vi "CTRE_CANTalonSRX_GetPID.vi"(0 "CAN Talon SRX Ref":T1={"DeviceStatus"={"status"=FALSE, "code"=0, "source"=""}, "Type"=enum."PWM", "PWM"={"PWM Channel"=enum."PWM 1", "DeadBand"={"Name"="", "maxPositivePwm"=0, "minPositivePwm"=0, "centerPwm"=0, "maxNegativePwm"=0, "minNegativePwm"=0, "angularRange"=0}}, "CAN"={"Device Number"=0, "SetOutput VI Ref"=variant(enum8{"Percent VBus", "Current", "Speed", "Position", "Voltage"} enum."Percent VBus"), "GetOutput VI Ref"=variant(refnum<k1> refnum), "Enable VI Ref"=variant(dbl 12.0), "Disable VI Ref"=variant(enum8{"Percent VBus", "Speed", "Position", "Slave", "Unchanged / Invalid", "Voltage Compensation", "Current", "Motion Profile"} enum."Percent VBus"), "Data"=variant}, "Invert"=FALSE}, 1 "Parameter Slot":u8 max=1, 11 "error in (no error)":errorcluster) -> (4 "CAN Talon SRX Ref":T1={"DeviceStatus"={"status"=FALSE, "code"=0, "source"=""}, "Type"=enum."PWM", "PWM"={"PWM Channel"=enum."PWM 1", "DeadBand"={"Name"="", "maxPositivePwm"=0, "minPositivePwm"=0, "centerPwm"=0, "maxNegativePwm"=0, "minNegativePwm"=0, "angularRange"=0}}, "CAN"={"Device Number"=0, "SetOutput VI Ref"=variant(enum8{"Percent VBus", "Current", "Speed", "Position", "Voltage"} enum."Percent VBus"), "GetOutput VI Ref"=variant(refnum<k1> refnum), "Enable VI Ref"=variant(dbl 12.0), "Disable VI Ref"=variant(enum8{"Percent VBus", "Speed", "Position", "Slave", "Unchanged / Invalid", "Voltage Compensation", "Current", "Motion Profile"} enum."Percent VBus"), "Data"=variant}, "Invert"=FALSE}, 6 "P":dbl, 8 "I":dbl, 10 "D":dbl, 12 "F":dbl, 13 "I Zone":dbl, 14 "Ramp Rate":dbl, 15 "error out":errorcluster)   [LabVIEW 2016]
doc: "Get the PID constants that are being used by the active parameter set on the Talon SRX.\n\nThis VI only applies in closed-loop modes."
uses:
  <vilib>/Rock Robotics/WPI/MotorControl/WPI_MotorControlDeviceRef.ctl
  <vilib>/Rock Robotics/WPI/MotorControl/WPI_MotorControlType.ctl
  <vilib>/Rock Robotics/SystemInterfaces/DIO/FPGA_DIOPWMChannel.ctl
  <vilib>/Rock Robotics/WPI/PWM/WPI_PWMDeadband.ctl
  <vilib>/Rock Robotics/WPI/ThirdParty/CanMotor/CTRLib-LV-TalonSRX/CTRE_CANTalonSRX_MessageIDs.ctl
  <vilib>/Rock Robotics/WPI/ThirdParty/CanMotor/CTRLib-LV-TalonSRX/CTRE_CANTalonSRX_Params.ctl
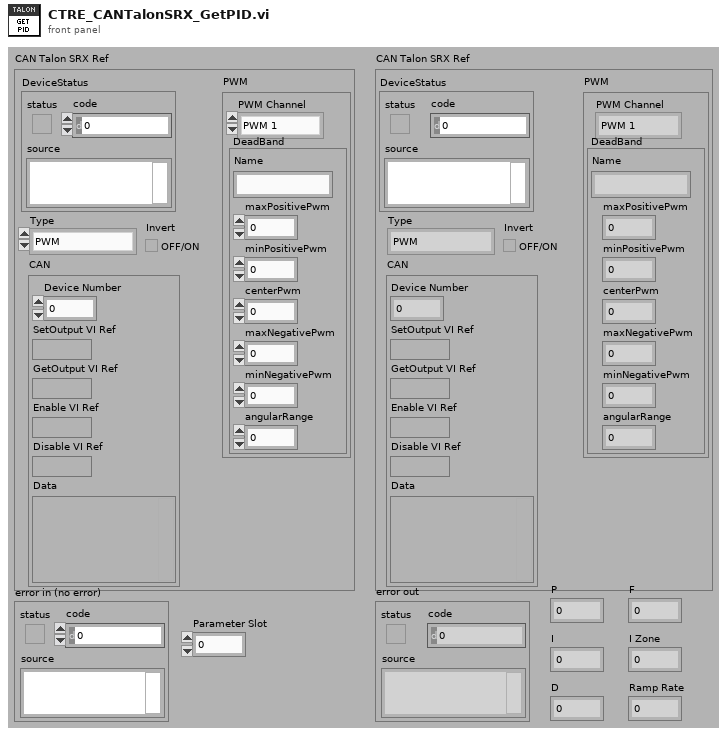
[diagram p1: front panel]
types:
  T1 = typedef "WPI_MotorControlDeviceRef.ctl" = cluster{"DeviceStatus":errorcluster, "Type":T2, "PWM":cluster{"PWM Channel":T3, "DeadBand":T4}, "CAN":cluster{"Device Number":u8, "SetOutput VI Ref":variant, "GetOutput VI Ref":variant, "Enable VI Ref":variant, "Disable VI Ref":variant, "Data":variant}, "Invert":bool}
  T2 = typedef "WPI_MotorControlType.ctl" = enum16{"PWM", "CAN"}
  T3 = typedef "FPGA_DIOPWMChannel.ctl" = enum8{"PWM 0", "PWM 1", "PWM 2", "PWM 3", "PWM 4", "PWM 5", "PWM 6", "PWM 7", "PWM 8", "PWM 9", "PWM MXP 0", "PWM MXP 1", "PWM MXP 2", "PWM MXP 3", "PWM MXP 4", "PWM MXP 5", "PWM MXP 6", "PWM MXP 7", "PWM MXP 8", "PWM MXP 9", "Invalid"}
  T4 = typedef "WPI_PWMDeadband.ctl" = cluster{"Name":string, "maxPositivePwm":i32, "minPositivePwm":i32, "centerPwm":i32, "maxNegativePwm":i32, "minNegativePwm":i32, "angularRange":u16}
  T5 = typedef "CTRE_CANTalonSRX_MessageIDs.ctl" = u32
  T6 = cluster{"Message ID":u32, "Timestamp":u32, "Data":u8[]}[]
  T7 = typedef "CTRE_CANTalonSRX_Params.ctl" = u8
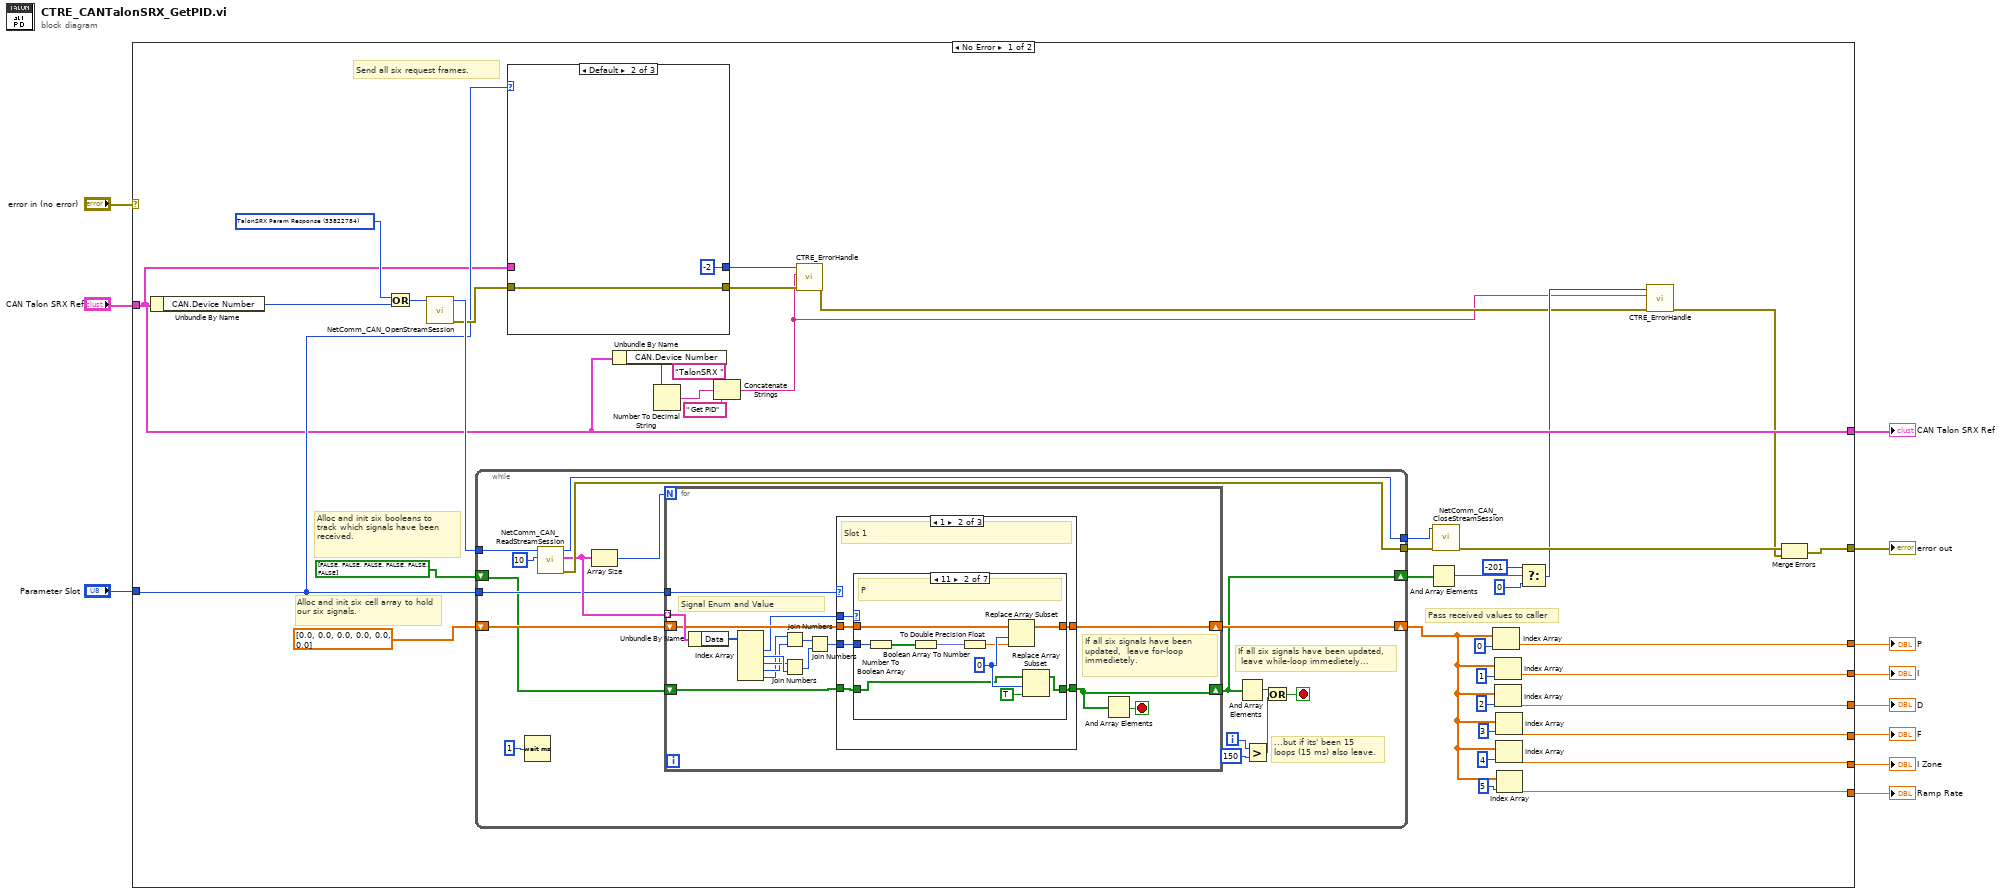
[diagram p0: block diagram]
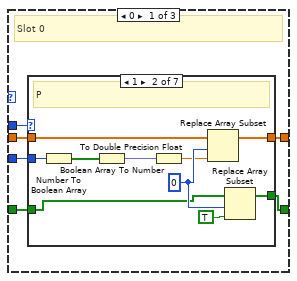
[diagram p2: hidden frame]
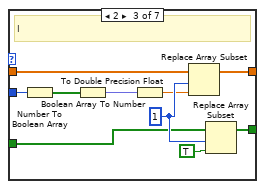
[diagram p4: hidden frame]
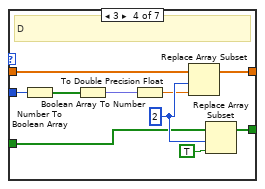
[diagram p5: hidden frame]
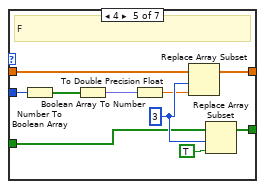
[diagram p6: hidden frame]
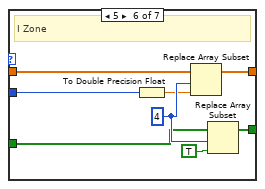
[diagram p7: hidden frame]
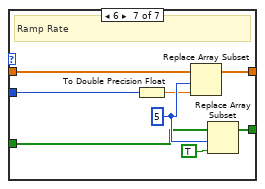
[diagram p8: hidden frame]
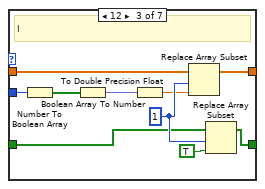
[diagram p10: hidden frame]
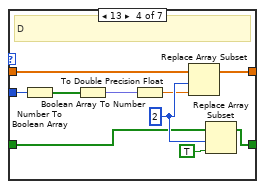
[diagram p11: hidden frame]
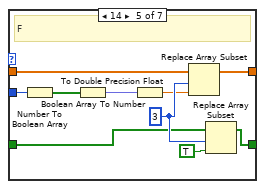
[diagram p12: hidden frame]
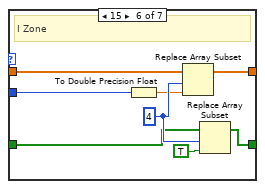
[diagram p13: hidden frame]
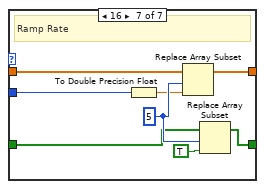
[diagram p14: hidden frame]
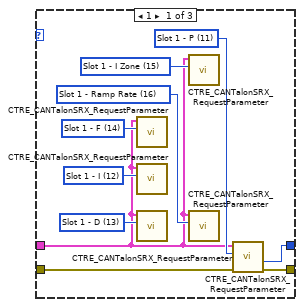
[diagram p16: hidden frame]
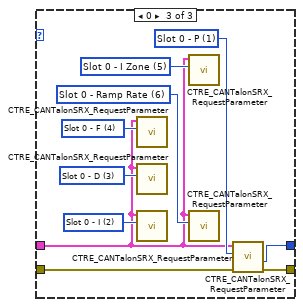
[diagram p17: hidden frame]
diagram:
  n1 = case shown="No Error" "error in (no error)" {
    selector: "error in (no error)" -> [_ w237]
    tunnel: [w19 w238] -> w11
    tunnel: "CAN Talon SRX Ref" -> [w19 w238]
    tunnel: [w27 w237] -> w9
    tunnel: "Parameter Slot" -> [w44 _]
    tunnel: [w42 _] -> w6
    tunnel: [w31 _] -> w5
    tunnel: [w36 _] -> w4
    tunnel: [w35 _] -> w3
    tunnel: [w34 _] -> w2
    tunnel: [w33 _] -> w1
    frame No Error {
      w51 = T5 33822784 items=["TalonSRX Control General 10ms"=33816576, "TalonSRX Control Rates Slow"=33816640, "TalonSRX Control ClearFlags Slow"=33816704, "TalonSRX Status General 10ms"=33821696, "TalonSRX Status Feedback 20ms"=33821760, "TalonSRX Status Enc 100ms"=33821824, "TalonSRX Status AinTempVbat 100ms"=33821888, "TalonSRX Status Startup Once"=33821952, "TalonSRX Status Debug"=33822080, "TalonSRX Config SetGainsSlot0 A"=33823808, "TalonSRX Config SetGainsSlot0 B"=33823872, "TalonSRX Config SetGainsSlot1 A"=33823936, "TalonSRX Config SetGainsSlot1 B"=33824000, "TalonSRX Config SetSoftLimits"=33824064, "TalonSRX Config WebControl"=33824128, "TalonSRX Param Request"=33822720, "TalonSRX Param Response"=33822784, "TalonSRX Param Set"=33822848]
      # "Pass received values to caller"
      # "Send all six request frames."
      # "Alloc and init six booleans to track which signals have been received."
      # "Alloc and init six cell array to hold our six signals."
      n2 = Unbundle By Name(w19) -> ("CAN.Device Number"=w50:u8)
      n3 = Or(x=w51, y=w50) -> (x .or. y?=w49:T5)
      n4 = call <vilib>:"NetComm_CAN_OpenStreamSession.vi"("Message ID"=w49) -> ("error out"=w45:errorcluster, "Session Handle"=w48:u32)  [unwired: 9 in]
      n5 = while {
        tunnel: [w65] -> w46
        tunnel: w48 -> [w68]
        tunnel: [w66] -> w47
        tunnel: w44 -> [w54]
        shift-right: [w57] -> w32
        shift-left: dbl[] [0.0, 0.0, 0.0, 0.0, 0.0, 0.0] ("Array") -> [w53]
        shift-right: [w55] -> w26
        shift-left: bool[] [FALSE, FALSE, FALSE, FALSE, FALSE, FALSE] ("Array") -> [w52]
        i -> [w63]
        stop <- w64 stop-if-true
        # "If all six signals have been updated,\n leave while-loop immedietely..."
        # "...but if its' been 15 \nloops (15 ms) also leave."
        n6 = Wait (ms)(milliseconds to wait=u32 1) -> ()  [unwired: 1 out]
        n7 = call <vilib>:"NetComm_CAN_ReadStreamSession.vi"("Messages To Read"=u32 10, "Session Handle"=w68) -> ("error out"=w65:errorcluster, "Messages"=w59:T6, "Session Handle Out"=w66:u32)  [unwired: 7 in]
        n8 = Array Size(array=w59) -> (size(s)=w56:i32)
        n9 = for {
          N: w56 -> [_]
          tunnel: w59 -> [w84] mode=indexing
          shift-right: [w72] -> w57
          shift-left: w53 -> [w74]
          shift-right: [w71] -> w55
          shift-left: w52 -> [w73]
          tunnel: w54 -> [w75]
          stop <- w76 stop-if-true
          # "Signal Enum and Value"
          # "If all six signals have been updated,  leave for-loop immedietely."
          n10 = Unbundle By Name(w84) -> ("Data"=w83:u8[])
          n11 = Index Array(array=w83) -> (element #1=w70:u8, element #2=w82:u8, element #3=w81:u8, element #4=w78:u8, element #5=w77:u8)  [unwired: 5 in]
          n12 = Join Numbers(hi=w77, lo=w78) -> ((hi.lo)=w79:u16)
          n13 = Join Numbers(hi=w81, lo=w82) -> ((hi.lo)=w80:u16)
          n14 = Join Numbers(hi=w79, lo=w80) -> ((hi.lo)=w69:u32)
          n15 = case shown="1" w75 {
            tunnel: w74 -> [w88 w154 w214]
            tunnel: w73 -> [w87 w153 w213]
            tunnel: [w85 w152 w214] -> w72
            tunnel: [w86 w151 w213] -> w71
            tunnel: w70 -> [w89 w150 _]
            tunnel: w69 -> [w90 w149 _]
            frame 0 {
              # "Slot 0"
              n16 = case shown="1" w89 {
                tunnel: [w92 w100 w107 w117 w127 w138 w144] -> w85
                tunnel: [w91 w97 w106 w116 w126 w136 w145] -> w86
                tunnel: w90 -> [_ w95 w103 w115 w125 w133 w141]
                tunnel: w88 -> [w92 w94 w105 w114 w124 w135 w142]
                tunnel: w87 -> [w91 w93 w104 w113 w123 w134 w143]
                frame Default {
                  # "Signal we don't care for"
                }
                frame 1 {
                  w98 = 0 ("index")
                  # "P"
                  n17 = Number To Boolean Array(number=w95) -> (Boolean array=w102:bool[])
                  n18 = Boolean Array To Number(Boolean array=w102) -> (number=w101:fxp<+,32,10>)
                  n19 = To Double Precision Float(number=w101) -> (double precision float=w96:dbl)
                  n20 = Replace Array Subset(array=w94, new element=w96, index=w98) -> (w100:dbl[])
                  n21 = Replace Array Subset(array=w93, new element=TRUE, index=w98) -> (w97:bool[])
                }
                frame 2 {
                  w109 = 1 ("index")
                  # "I"
                  n22 = Number To Boolean Array(number=w103) -> (Boolean array=w112:bool[])
                  n23 = Boolean Array To Number(Boolean array=w112) -> (number=w111:fxp<+,32,10>)
                  n24 = To Double Precision Float(number=w111) -> (double precision float=w108:dbl)
                  n25 = Replace Array Subset(array=w105, new element=w108, index=w109) -> (w107:dbl[])
                  n26 = Replace Array Subset(array=w104, new element=TRUE, index=w109) -> (w106:bool[])
                }
                frame 3 {
                  w119 = 2 ("index")
                  # "D"
                  n27 = Number To Boolean Array(number=w115) -> (Boolean array=w122:bool[])
                  n28 = Boolean Array To Number(Boolean array=w122) -> (number=w121:fxp<+,32,10>)
                  n29 = To Double Precision Float(number=w121) -> (double precision float=w118:dbl)
                  n30 = Replace Array Subset(array=w114, new element=w118, index=w119) -> (w117:dbl[])
                  n31 = Replace Array Subset(array=w113, new element=TRUE, index=w119) -> (w116:bool[])
                }
                frame 4 {
                  w129 = 3 ("index")
                  # "F"
                  n32 = Number To Boolean Array(number=w125) -> (Boolean array=w132:bool[])
                  n33 = Boolean Array To Number(Boolean array=w132) -> (number=w131:fxp<+/-,32,10>)
                  n34 = To Double Precision Float(number=w131) -> (double precision float=w128:dbl)
                  n35 = Replace Array Subset(array=w124, new element=w128, index=w129) -> (w127:dbl[])
                  n36 = Replace Array Subset(array=w123, new element=TRUE, index=w129) -> (w126:bool[])
                }
                frame 5 {
                  w139 = 4 ("index")
                  # "I Zone"
                  n37 = To Double Precision Float(number=w133) -> (double precision float=w137:dbl)
                  n38 = Replace Array Subset(array=w135, new element=w137, index=w139) -> (w138:dbl[])
                  n39 = Replace Array Subset(array=w134, new element=TRUE, index=w139) -> (w136:bool[])
                }
                frame 6 {
                  w147 = 5 ("index")
                  # "Ramp Rate"
                  n40 = To Double Precision Float(number=w141) -> (double precision float=w146:dbl)
                  n41 = Replace Array Subset(array=w142, new element=w146, index=w147) -> (w144:dbl[])
                  n42 = Replace Array Subset(array=w143, new element=TRUE, index=w147) -> (w145:bool[])
                }
              }
            }
            frame 1 {
              # "Slot 1"
              n43 = case shown="11" w150 {
                tunnel: w149 -> [_ w166 w176 w186 w196 w204 w212]
                tunnel: w154 -> [w155 w163 w170 w177 w189 w199 w208]
                tunnel: [w155 w162 w169 w180 w190 w201 w205] -> w152
                tunnel: w153 -> [w156 w159 w167 w178 w188 w198 w207]
                tunnel: [w156 w158 w168 w179 w187 w197 w206] -> w151
                frame Default {
                  # "Signal we don't care for"
                }
                frame 11 {
                  w160 = 0 ("index")
                  # "P"
                  n44 = Number To Boolean Array(number=w166) -> (Boolean array=w165:bool[])
                  n45 = Boolean Array To Number(Boolean array=w165) -> (number=w164:fxp<+,32,10>)
                  n46 = To Double Precision Float(number=w164) -> (double precision float=w157:dbl)
                  n47 = Replace Array Subset(array=w163, new element=w157, index=w160) -> (w162:dbl[])
                  n48 = Replace Array Subset(array=w159, new element=TRUE, index=w160) -> (w158:bool[])
                }
                frame 12 {
                  w172 = 1 ("index")
                  # "I"
                  n49 = Number To Boolean Array(number=w176) -> (Boolean array=w175:bool[])
                  n50 = Boolean Array To Number(Boolean array=w175) -> (number=w174:fxp<+,32,10>)
                  n51 = To Double Precision Float(number=w174) -> (double precision float=w171:dbl)
                  n52 = Replace Array Subset(array=w170, new element=w171, index=w172) -> (w169:dbl[])
                  n53 = Replace Array Subset(array=w167, new element=TRUE, index=w172) -> (w168:bool[])
                }
                frame 13 {
                  w182 = 2 ("index")
                  # "D"
                  n54 = Number To Boolean Array(number=w186) -> (Boolean array=w185:bool[])
                  n55 = Boolean Array To Number(Boolean array=w185) -> (number=w184:fxp<+,32,10>)
                  n56 = To Double Precision Float(number=w184) -> (double precision float=w181:dbl)
                  n57 = Replace Array Subset(array=w177, new element=w181, index=w182) -> (w180:dbl[])
                  n58 = Replace Array Subset(array=w178, new element=TRUE, index=w182) -> (w179:bool[])
                }
                frame 14 {
                  w192 = 3 ("index")
                  # "F"
                  n59 = Number To Boolean Array(number=w196) -> (Boolean array=w195:bool[])
                  n60 = Boolean Array To Number(Boolean array=w195) -> (number=w194:fxp<+/-,32,10>)
                  n61 = To Double Precision Float(number=w194) -> (double precision float=w191:dbl)
                  n62 = Replace Array Subset(array=w189, new element=w191, index=w192) -> (w190:dbl[])
                  n63 = Replace Array Subset(array=w188, new element=TRUE, index=w192) -> (w187:bool[])
                }
                frame 15 {
                  w202 = 4 ("index")
                  # "I Zone"
                  n64 = To Double Precision Float(number=w204) -> (double precision float=w200:dbl)
                  n65 = Replace Array Subset(array=w199, new element=w200, index=w202) -> (w201:dbl[])
                  n66 = Replace Array Subset(array=w198, new element=TRUE, index=w202) -> (w197:bool[])
                }
                frame 16 {
                  w210 = 5 ("index")
                  # "Ramp Rate"
                  n67 = To Double Precision Float(number=w212) -> (double precision float=w209:dbl)
                  n68 = Replace Array Subset(array=w208, new element=w209, index=w210) -> (w205:dbl[])
                  n69 = Replace Array Subset(array=w207, new element=TRUE, index=w210) -> (w206:bool[])
                }
              }
            }
            frame Default {
              # "Invalid Slot"
            }
          }
          n70 = And Array Elements(Boolean array=w71) -> (logical AND=w76:bool)
        }
        n71 = And Array Elements(Boolean array=w55) -> (logical AND=w58:bool)
        n72 = Greater?(x=w63, y=150) -> (0:w60:bool)
        n73 = Or(x=w58, y=w60) -> (x .or. y?=w64:bool)
      }
      n74 = case shown="Default" w44 {
        tunnel: [w218 w226 w235] -> w25
        tunnel: w45 -> [w217 w226 w229]
        tunnel: w19 -> [w216 _ w228]
        tunnel: [w215 -2 ("Code") w227] -> w24
        frame 1 {
          w223 = T7 16 items=["Slot 0 - P"=1, "Slot 0 - I"=2, "Slot 0 - D"=3, "Slot 0 - F"=4, "Slot 0 - I Zone"=5, "Slot 0 - Ramp Rate"=6, "Slot 1 - P"=11, "Slot 1 - I"=12, "Slot 1 - D"=13, "Slot 1 - F"=14, "Slot 1 - I Zone"=15, "Slot 1 - Ramp Rate"=16, "Soft Limit - Forward"=21, "Soft Limit - Reverse"=22, "On Boot - Brake Mode"=31, "On Boot - Limit Normally Closed - Forward"=32, "On Boot - Limit Normally Closed - Reverse"=33, "On Boot - Limit Disabled - Forward"=34, "On Boot - Limit Disabled - Reverse"=35, "Fault - Over Temp"=41, "Fault - Under Voltage"=42, "Fault - Forward Limit"=43, "Fault - Reverse Limit"=44, "Fault - Hardware Failure"=45, "Fault - Forward Soft Limit"=46, "Fault - Reverse Soft Limit"=47, "Sticky Fault - Over Temp"=48, "Sticky Fault - Under Voltage"=49, "Sticky Fault - Forward Limit"=50, "Sticky Fault - Reverse Limit"=51, "Sticky Fault - Forward Soft Limit"=52, "Sticky Fault - Reverse Soft Limit"=53, "Applied Throttle"=61, "Closed-Loop Error"=62, "Select Feedback Device"=63, "Reverse Closed-Loop Output"=64, "Mode Select"=65, "Profile Slot Select"=66, "Ramp Throttle"=67, "Reverse Feedback Sensor"=68, "Limit Switch Enabled"=69, "Limit Switch Closed - Forward"=70, "Limit Switch Closed - Reverse"=71, "Sensor Position"=73, "Sensor Velocity"=74, "Current"=75, "Brake is Enabled"=76, "Encoder Position"=77, "Encoder Velocity"=78, "Encoder Index Rise Events"=79, "Encoder A Pin State"=80, "Encoder B Pin State"=81, "Encoder Index Pin State"=82, "Analog In with Overflow"=83, "Analog In Velocity"=84, "Temperature"=85, "Battery Voltage"=86, "Reset Count"=87, "Reset Flags"=88, "Firmware Version"=89, "Settings Changed"=90] ("Parameter")
          w222 = T7 15 items=["Slot 0 - P"=1, "Slot 0 - I"=2, "Slot 0 - D"=3, "Slot 0 - F"=4, "Slot 0 - I Zone"=5, "Slot 0 - Ramp Rate"=6, "Slot 1 - P"=11, "Slot 1 - I"=12, "Slot 1 - D"=13, "Slot 1 - F"=14, "Slot 1 - I Zone"=15, "Slot 1 - Ramp Rate"=16, "Soft Limit - Forward"=21, "Soft Limit - Reverse"=22, "On Boot - Brake Mode"=31, "On Boot - Limit Normally Closed - Forward"=32, "On Boot - Limit Normally Closed - Reverse"=33, "On Boot - Limit Disabled - Forward"=34, "On Boot - Limit Disabled - Reverse"=35, "Fault - Over Temp"=41, "Fault - Under Voltage"=42, "Fault - Forward Limit"=43, "Fault - Reverse Limit"=44, "Fault - Hardware Failure"=45, "Fault - Forward Soft Limit"=46, "Fault - Reverse Soft Limit"=47, "Sticky Fault - Over Temp"=48, "Sticky Fault - Under Voltage"=49, "Sticky Fault - Forward Limit"=50, "Sticky Fault - Reverse Limit"=51, "Sticky Fault - Forward Soft Limit"=52, "Sticky Fault - Reverse Soft Limit"=53, "Applied Throttle"=61, "Closed-Loop Error"=62, "Select Feedback Device"=63, "Reverse Closed-Loop Output"=64, "Mode Select"=65, "Profile Slot Select"=66, "Ramp Throttle"=67, "Reverse Feedback Sensor"=68, "Limit Switch Enabled"=69, "Limit Switch Closed - Forward"=70, "Limit Switch Closed - Reverse"=71, "Sensor Position"=73, "Sensor Velocity"=74, "Current"=75, "Brake is Enabled"=76, "Encoder Position"=77, "Encoder Velocity"=78, "Encoder Index Rise Events"=79, "Encoder A Pin State"=80, "Encoder B Pin State"=81, "Encoder Index Pin State"=82, "Analog In with Overflow"=83, "Analog In Velocity"=84, "Temperature"=85, "Battery Voltage"=86, "Reset Count"=87, "Reset Flags"=88, "Firmware Version"=89, "Settings Changed"=90] ("Parameter")
          w221 = T7 14 items=["Slot 0 - P"=1, "Slot 0 - I"=2, "Slot 0 - D"=3, "Slot 0 - F"=4, "Slot 0 - I Zone"=5, "Slot 0 - Ramp Rate"=6, "Slot 1 - P"=11, "Slot 1 - I"=12, "Slot 1 - D"=13, "Slot 1 - F"=14, "Slot 1 - I Zone"=15, "Slot 1 - Ramp Rate"=16, "Soft Limit - Forward"=21, "Soft Limit - Reverse"=22, "On Boot - Brake Mode"=31, "On Boot - Limit Normally Closed - Forward"=32, "On Boot - Limit Normally Closed - Reverse"=33, "On Boot - Limit Disabled - Forward"=34, "On Boot - Limit Disabled - Reverse"=35, "Fault - Over Temp"=41, "Fault - Under Voltage"=42, "Fault - Forward Limit"=43, "Fault - Reverse Limit"=44, "Fault - Hardware Failure"=45, "Fault - Forward Soft Limit"=46, "Fault - Reverse Soft Limit"=47, "Sticky Fault - Over Temp"=48, "Sticky Fault - Under Voltage"=49, "Sticky Fault - Forward Limit"=50, "Sticky Fault - Reverse Limit"=51, "Sticky Fault - Forward Soft Limit"=52, "Sticky Fault - Reverse Soft Limit"=53, "Applied Throttle"=61, "Closed-Loop Error"=62, "Select Feedback Device"=63, "Reverse Closed-Loop Output"=64, "Mode Select"=65, "Profile Slot Select"=66, "Ramp Throttle"=67, "Reverse Feedback Sensor"=68, "Limit Switch Enabled"=69, "Limit Switch Closed - Forward"=70, "Limit Switch Closed - Reverse"=71, "Sensor Position"=73, "Sensor Velocity"=74, "Current"=75, "Brake is Enabled"=76, "Encoder Position"=77, "Encoder Velocity"=78, "Encoder Index Rise Events"=79, "Encoder A Pin State"=80, "Encoder B Pin State"=81, "Encoder Index Pin State"=82, "Analog In with Overflow"=83, "Analog In Velocity"=84, "Temperature"=85, "Battery Voltage"=86, "Reset Count"=87, "Reset Flags"=88, "Firmware Version"=89, "Settings Changed"=90] ("Parameter")
          w220 = T7 13 items=["Slot 0 - P"=1, "Slot 0 - I"=2, "Slot 0 - D"=3, "Slot 0 - F"=4, "Slot 0 - I Zone"=5, "Slot 0 - Ramp Rate"=6, "Slot 1 - P"=11, "Slot 1 - I"=12, "Slot 1 - D"=13, "Slot 1 - F"=14, "Slot 1 - I Zone"=15, "Slot 1 - Ramp Rate"=16, "Soft Limit - Forward"=21, "Soft Limit - Reverse"=22, "On Boot - Brake Mode"=31, "On Boot - Limit Normally Closed - Forward"=32, "On Boot - Limit Normally Closed - Reverse"=33, "On Boot - Limit Disabled - Forward"=34, "On Boot - Limit Disabled - Reverse"=35, "Fault - Over Temp"=41, "Fault - Under Voltage"=42, "Fault - Forward Limit"=43, "Fault - Reverse Limit"=44, "Fault - Hardware Failure"=45, "Fault - Forward Soft Limit"=46, "Fault - Reverse Soft Limit"=47, "Sticky Fault - Over Temp"=48, "Sticky Fault - Under Voltage"=49, "Sticky Fault - Forward Limit"=50, "Sticky Fault - Reverse Limit"=51, "Sticky Fault - Forward Soft Limit"=52, "Sticky Fault - Reverse Soft Limit"=53, "Applied Throttle"=61, "Closed-Loop Error"=62, "Select Feedback Device"=63, "Reverse Closed-Loop Output"=64, "Mode Select"=65, "Profile Slot Select"=66, "Ramp Throttle"=67, "Reverse Feedback Sensor"=68, "Limit Switch Enabled"=69, "Limit Switch Closed - Forward"=70, "Limit Switch Closed - Reverse"=71, "Sensor Position"=73, "Sensor Velocity"=74, "Current"=75, "Brake is Enabled"=76, "Encoder Position"=77, "Encoder Velocity"=78, "Encoder Index Rise Events"=79, "Encoder A Pin State"=80, "Encoder B Pin State"=81, "Encoder Index Pin State"=82, "Analog In with Overflow"=83, "Analog In Velocity"=84, "Temperature"=85, "Battery Voltage"=86, "Reset Count"=87, "Reset Flags"=88, "Firmware Version"=89, "Settings Changed"=90] ("Parameter")
          w219 = T7 12 items=["Slot 0 - P"=1, "Slot 0 - I"=2, "Slot 0 - D"=3, "Slot 0 - F"=4, "Slot 0 - I Zone"=5, "Slot 0 - Ramp Rate"=6, "Slot 1 - P"=11, "Slot 1 - I"=12, "Slot 1 - D"=13, "Slot 1 - F"=14, "Slot 1 - I Zone"=15, "Slot 1 - Ramp Rate"=16, "Soft Limit - Forward"=21, "Soft Limit - Reverse"=22, "On Boot - Brake Mode"=31, "On Boot - Limit Normally Closed - Forward"=32, "On Boot - Limit Normally Closed - Reverse"=33, "On Boot - Limit Disabled - Forward"=34, "On Boot - Limit Disabled - Reverse"=35, "Fault - Over Temp"=41, "Fault - Under Voltage"=42, "Fault - Forward Limit"=43, "Fault - Reverse Limit"=44, "Fault - Hardware Failure"=45, "Fault - Forward Soft Limit"=46, "Fault - Reverse Soft Limit"=47, "Sticky Fault - Over Temp"=48, "Sticky Fault - Under Voltage"=49, "Sticky Fault - Forward Limit"=50, "Sticky Fault - Reverse Limit"=51, "Sticky Fault - Forward Soft Limit"=52, "Sticky Fault - Reverse Soft Limit"=53, "Applied Throttle"=61, "Closed-Loop Error"=62, "Select Feedback Device"=63, "Reverse Closed-Loop Output"=64, "Mode Select"=65, "Profile Slot Select"=66, "Ramp Throttle"=67, "Reverse Feedback Sensor"=68, "Limit Switch Enabled"=69, "Limit Switch Closed - Forward"=70, "Limit Switch Closed - Reverse"=71, "Sensor Position"=73, "Sensor Velocity"=74, "Current"=75, "Brake is Enabled"=76, "Encoder Position"=77, "Encoder Velocity"=78, "Encoder Index Rise Events"=79, "Encoder A Pin State"=80, "Encoder B Pin State"=81, "Encoder Index Pin State"=82, "Analog In with Overflow"=83, "Analog In Velocity"=84, "Temperature"=85, "Battery Voltage"=86, "Reset Count"=87, "Reset Flags"=88, "Firmware Version"=89, "Settings Changed"=90] ("Parameter")
          w224 = T7 11 items=["Slot 0 - P"=1, "Slot 0 - I"=2, "Slot 0 - D"=3, "Slot 0 - F"=4, "Slot 0 - I Zone"=5, "Slot 0 - Ramp Rate"=6, "Slot 1 - P"=11, "Slot 1 - I"=12, "Slot 1 - D"=13, "Slot 1 - F"=14, "Slot 1 - I Zone"=15, "Slot 1 - Ramp Rate"=16, "Soft Limit - Forward"=21, "Soft Limit - Reverse"=22, "On Boot - Brake Mode"=31, "On Boot - Limit Normally Closed - Forward"=32, "On Boot - Limit Normally Closed - Reverse"=33, "On Boot - Limit Disabled - Forward"=34, "On Boot - Limit Disabled - Reverse"=35, "Fault - Over Temp"=41, "Fault - Under Voltage"=42, "Fault - Forward Limit"=43, "Fault - Reverse Limit"=44, "Fault - Hardware Failure"=45, "Fault - Forward Soft Limit"=46, "Fault - Reverse Soft Limit"=47, "Sticky Fault - Over Temp"=48, "Sticky Fault - Under Voltage"=49, "Sticky Fault - Forward Limit"=50, "Sticky Fault - Reverse Limit"=51, "Sticky Fault - Forward Soft Limit"=52, "Sticky Fault - Reverse Soft Limit"=53, "Applied Throttle"=61, "Closed-Loop Error"=62, "Select Feedback Device"=63, "Reverse Closed-Loop Output"=64, "Mode Select"=65, "Profile Slot Select"=66, "Ramp Throttle"=67, "Reverse Feedback Sensor"=68, "Limit Switch Enabled"=69, "Limit Switch Closed - Forward"=70, "Limit Switch Closed - Reverse"=71, "Sensor Position"=73, "Sensor Velocity"=74, "Current"=75, "Brake is Enabled"=76, "Encoder Position"=77, "Encoder Velocity"=78, "Encoder Index Rise Events"=79, "Encoder A Pin State"=80, "Encoder B Pin State"=81, "Encoder Index Pin State"=82, "Analog In with Overflow"=83, "Analog In Velocity"=84, "Temperature"=85, "Battery Voltage"=86, "Reset Count"=87, "Reset Flags"=88, "Firmware Version"=89, "Settings Changed"=90] ("Parameter")
          n75 = call <vilib>:"CTRE_CANTalonSRX_RequestParameter.vi"("Parameter"=w221, "CAN Talon SRX Ref"=w216) -> ()  [unwired: 7 in, 3 out]
          n76 = call <vilib>:"CTRE_CANTalonSRX_RequestParameter.vi"("Parameter"=w219, "CAN Talon SRX Ref"=w216) -> ()  [unwired: 7 in, 3 out]
          n77 = call <vilib>:"CTRE_CANTalonSRX_RequestParameter.vi"("Parameter"=w220, "CAN Talon SRX Ref"=w216) -> ()  [unwired: 7 in, 3 out]
          n78 = call <vilib>:"CTRE_CANTalonSRX_RequestParameter.vi"("Parameter"=w222, "CAN Talon SRX Ref"=w216) -> ()  [unwired: 7 in, 3 out]
          n79 = call <vilib>:"CTRE_CANTalonSRX_RequestParameter.vi"("Parameter"=w223, "CAN Talon SRX Ref"=w216) -> ()  [unwired: 7 in, 3 out]
          n80 = call <vilib>:"CTRE_CANTalonSRX_RequestParameter.vi"("error in (no error)"=w217, "Parameter"=w224, "CAN Talon SRX Ref"=w216) -> ("error out"=w218:errorcluster, "Code"=w215:i32)  [unwired: 6 in, 1 out]
        }
        frame Default {
        }
        frame 0 {
          w233 = T7 6 items=["Slot 0 - P"=1, "Slot 0 - I"=2, "Slot 0 - D"=3, "Slot 0 - F"=4, "Slot 0 - I Zone"=5, "Slot 0 - Ramp Rate"=6, "Slot 1 - P"=11, "Slot 1 - I"=12, "Slot 1 - D"=13, "Slot 1 - F"=14, "Slot 1 - I Zone"=15, "Slot 1 - Ramp Rate"=16, "Soft Limit - Forward"=21, "Soft Limit - Reverse"=22, "On Boot - Brake Mode"=31, "On Boot - Limit Normally Closed - Forward"=32, "On Boot - Limit Normally Closed - Reverse"=33, "On Boot - Limit Disabled - Forward"=34, "On Boot - Limit Disabled - Reverse"=35, "Fault - Over Temp"=41, "Fault - Under Voltage"=42, "Fault - Forward Limit"=43, "Fault - Reverse Limit"=44, "Fault - Hardware Failure"=45, "Fault - Forward Soft Limit"=46, "Fault - Reverse Soft Limit"=47, "Sticky Fault - Over Temp"=48, "Sticky Fault - Under Voltage"=49, "Sticky Fault - Forward Limit"=50, "Sticky Fault - Reverse Limit"=51, "Sticky Fault - Forward Soft Limit"=52, "Sticky Fault - Reverse Soft Limit"=53, "Applied Throttle"=61, "Closed-Loop Error"=62, "Select Feedback Device"=63, "Reverse Closed-Loop Output"=64, "Mode Select"=65, "Profile Slot Select"=66, "Ramp Throttle"=67, "Reverse Feedback Sensor"=68, "Limit Switch Enabled"=69, "Limit Switch Closed - Forward"=70, "Limit Switch Closed - Reverse"=71, "Sensor Position"=73, "Sensor Velocity"=74, "Current"=75, "Brake is Enabled"=76, "Encoder Position"=77, "Encoder Velocity"=78, "Encoder Index Rise Events"=79, "Encoder A Pin State"=80, "Encoder B Pin State"=81, "Encoder Index Pin State"=82, "Analog In with Overflow"=83, "Analog In Velocity"=84, "Temperature"=85, "Battery Voltage"=86, "Reset Count"=87, "Reset Flags"=88, "Firmware Version"=89, "Settings Changed"=90] ("Parameter")
          w232 = T7 5 items=["Slot 0 - P"=1, "Slot 0 - I"=2, "Slot 0 - D"=3, "Slot 0 - F"=4, "Slot 0 - I Zone"=5, "Slot 0 - Ramp Rate"=6, "Slot 1 - P"=11, "Slot 1 - I"=12, "Slot 1 - D"=13, "Slot 1 - F"=14, "Slot 1 - I Zone"=15, "Slot 1 - Ramp Rate"=16, "Soft Limit - Forward"=21, "Soft Limit - Reverse"=22, "On Boot - Brake Mode"=31, "On Boot - Limit Normally Closed - Forward"=32, "On Boot - Limit Normally Closed - Reverse"=33, "On Boot - Limit Disabled - Forward"=34, "On Boot - Limit Disabled - Reverse"=35, "Fault - Over Temp"=41, "Fault - Under Voltage"=42, "Fault - Forward Limit"=43, "Fault - Reverse Limit"=44, "Fault - Hardware Failure"=45, "Fault - Forward Soft Limit"=46, "Fault - Reverse Soft Limit"=47, "Sticky Fault - Over Temp"=48, "Sticky Fault - Under Voltage"=49, "Sticky Fault - Forward Limit"=50, "Sticky Fault - Reverse Limit"=51, "Sticky Fault - Forward Soft Limit"=52, "Sticky Fault - Reverse Soft Limit"=53, "Applied Throttle"=61, "Closed-Loop Error"=62, "Select Feedback Device"=63, "Reverse Closed-Loop Output"=64, "Mode Select"=65, "Profile Slot Select"=66, "Ramp Throttle"=67, "Reverse Feedback Sensor"=68, "Limit Switch Enabled"=69, "Limit Switch Closed - Forward"=70, "Limit Switch Closed - Reverse"=71, "Sensor Position"=73, "Sensor Velocity"=74, "Current"=75, "Brake is Enabled"=76, "Encoder Position"=77, "Encoder Velocity"=78, "Encoder Index Rise Events"=79, "Encoder A Pin State"=80, "Encoder B Pin State"=81, "Encoder Index Pin State"=82, "Analog In with Overflow"=83, "Analog In Velocity"=84, "Temperature"=85, "Battery Voltage"=86, "Reset Count"=87, "Reset Flags"=88, "Firmware Version"=89, "Settings Changed"=90] ("Parameter")
          w231 = T7 4 items=["Slot 0 - P"=1, "Slot 0 - I"=2, "Slot 0 - D"=3, "Slot 0 - F"=4, "Slot 0 - I Zone"=5, "Slot 0 - Ramp Rate"=6, "Slot 1 - P"=11, "Slot 1 - I"=12, "Slot 1 - D"=13, "Slot 1 - F"=14, "Slot 1 - I Zone"=15, "Slot 1 - Ramp Rate"=16, "Soft Limit - Forward"=21, "Soft Limit - Reverse"=22, "On Boot - Brake Mode"=31, "On Boot - Limit Normally Closed - Forward"=32, "On Boot - Limit Normally Closed - Reverse"=33, "On Boot - Limit Disabled - Forward"=34, "On Boot - Limit Disabled - Reverse"=35, "Fault - Over Temp"=41, "Fault - Under Voltage"=42, "Fault - Forward Limit"=43, "Fault - Reverse Limit"=44, "Fault - Hardware Failure"=45, "Fault - Forward Soft Limit"=46, "Fault - Reverse Soft Limit"=47, "Sticky Fault - Over Temp"=48, "Sticky Fault - Under Voltage"=49, "Sticky Fault - Forward Limit"=50, "Sticky Fault - Reverse Limit"=51, "Sticky Fault - Forward Soft Limit"=52, "Sticky Fault - Reverse Soft Limit"=53, "Applied Throttle"=61, "Closed-Loop Error"=62, "Select Feedback Device"=63, "Reverse Closed-Loop Output"=64, "Mode Select"=65, "Profile Slot Select"=66, "Ramp Throttle"=67, "Reverse Feedback Sensor"=68, "Limit Switch Enabled"=69, "Limit Switch Closed - Forward"=70, "Limit Switch Closed - Reverse"=71, "Sensor Position"=73, "Sensor Velocity"=74, "Current"=75, "Brake is Enabled"=76, "Encoder Position"=77, "Encoder Velocity"=78, "Encoder Index Rise Events"=79, "Encoder A Pin State"=80, "Encoder B Pin State"=81, "Encoder Index Pin State"=82, "Analog In with Overflow"=83, "Analog In Velocity"=84, "Temperature"=85, "Battery Voltage"=86, "Reset Count"=87, "Reset Flags"=88, "Firmware Version"=89, "Settings Changed"=90] ("Parameter")
          w230 = T7 3 items=["Slot 0 - P"=1, "Slot 0 - I"=2, "Slot 0 - D"=3, "Slot 0 - F"=4, "Slot 0 - I Zone"=5, "Slot 0 - Ramp Rate"=6, "Slot 1 - P"=11, "Slot 1 - I"=12, "Slot 1 - D"=13, "Slot 1 - F"=14, "Slot 1 - I Zone"=15, "Slot 1 - Ramp Rate"=16, "Soft Limit - Forward"=21, "Soft Limit - Reverse"=22, "On Boot - Brake Mode"=31, "On Boot - Limit Normally Closed - Forward"=32, "On Boot - Limit Normally Closed - Reverse"=33, "On Boot - Limit Disabled - Forward"=34, "On Boot - Limit Disabled - Reverse"=35, "Fault - Over Temp"=41, "Fault - Under Voltage"=42, "Fault - Forward Limit"=43, "Fault - Reverse Limit"=44, "Fault - Hardware Failure"=45, "Fault - Forward Soft Limit"=46, "Fault - Reverse Soft Limit"=47, "Sticky Fault - Over Temp"=48, "Sticky Fault - Under Voltage"=49, "Sticky Fault - Forward Limit"=50, "Sticky Fault - Reverse Limit"=51, "Sticky Fault - Forward Soft Limit"=52, "Sticky Fault - Reverse Soft Limit"=53, "Applied Throttle"=61, "Closed-Loop Error"=62, "Select Feedback Device"=63, "Reverse Closed-Loop Output"=64, "Mode Select"=65, "Profile Slot Select"=66, "Ramp Throttle"=67, "Reverse Feedback Sensor"=68, "Limit Switch Enabled"=69, "Limit Switch Closed - Forward"=70, "Limit Switch Closed - Reverse"=71, "Sensor Position"=73, "Sensor Velocity"=74, "Current"=75, "Brake is Enabled"=76, "Encoder Position"=77, "Encoder Velocity"=78, "Encoder Index Rise Events"=79, "Encoder A Pin State"=80, "Encoder B Pin State"=81, "Encoder Index Pin State"=82, "Analog In with Overflow"=83, "Analog In Velocity"=84, "Temperature"=85, "Battery Voltage"=86, "Reset Count"=87, "Reset Flags"=88, "Firmware Version"=89, "Settings Changed"=90] ("Parameter")
          w234 = T7 2 items=["Slot 0 - P"=1, "Slot 0 - I"=2, "Slot 0 - D"=3, "Slot 0 - F"=4, "Slot 0 - I Zone"=5, "Slot 0 - Ramp Rate"=6, "Slot 1 - P"=11, "Slot 1 - I"=12, "Slot 1 - D"=13, "Slot 1 - F"=14, "Slot 1 - I Zone"=15, "Slot 1 - Ramp Rate"=16, "Soft Limit - Forward"=21, "Soft Limit - Reverse"=22, "On Boot - Brake Mode"=31, "On Boot - Limit Normally Closed - Forward"=32, "On Boot - Limit Normally Closed - Reverse"=33, "On Boot - Limit Disabled - Forward"=34, "On Boot - Limit Disabled - Reverse"=35, "Fault - Over Temp"=41, "Fault - Under Voltage"=42, "Fault - Forward Limit"=43, "Fault - Reverse Limit"=44, "Fault - Hardware Failure"=45, "Fault - Forward Soft Limit"=46, "Fault - Reverse Soft Limit"=47, "Sticky Fault - Over Temp"=48, "Sticky Fault - Under Voltage"=49, "Sticky Fault - Forward Limit"=50, "Sticky Fault - Reverse Limit"=51, "Sticky Fault - Forward Soft Limit"=52, "Sticky Fault - Reverse Soft Limit"=53, "Applied Throttle"=61, "Closed-Loop Error"=62, "Select Feedback Device"=63, "Reverse Closed-Loop Output"=64, "Mode Select"=65, "Profile Slot Select"=66, "Ramp Throttle"=67, "Reverse Feedback Sensor"=68, "Limit Switch Enabled"=69, "Limit Switch Closed - Forward"=70, "Limit Switch Closed - Reverse"=71, "Sensor Position"=73, "Sensor Velocity"=74, "Current"=75, "Brake is Enabled"=76, "Encoder Position"=77, "Encoder Velocity"=78, "Encoder Index Rise Events"=79, "Encoder A Pin State"=80, "Encoder B Pin State"=81, "Encoder Index Pin State"=82, "Analog In with Overflow"=83, "Analog In Velocity"=84, "Temperature"=85, "Battery Voltage"=86, "Reset Count"=87, "Reset Flags"=88, "Firmware Version"=89, "Settings Changed"=90] ("Parameter")
          w236 = T7 1 items=["Slot 0 - P"=1, "Slot 0 - I"=2, "Slot 0 - D"=3, "Slot 0 - F"=4, "Slot 0 - I Zone"=5, "Slot 0 - Ramp Rate"=6, "Slot 1 - P"=11, "Slot 1 - I"=12, "Slot 1 - D"=13, "Slot 1 - F"=14, "Slot 1 - I Zone"=15, "Slot 1 - Ramp Rate"=16, "Soft Limit - Forward"=21, "Soft Limit - Reverse"=22, "On Boot - Brake Mode"=31, "On Boot - Limit Normally Closed - Forward"=32, "On Boot - Limit Normally Closed - Reverse"=33, "On Boot - Limit Disabled - Forward"=34, "On Boot - Limit Disabled - Reverse"=35, "Fault - Over Temp"=41, "Fault - Under Voltage"=42, "Fault - Forward Limit"=43, "Fault - Reverse Limit"=44, "Fault - Hardware Failure"=45, "Fault - Forward Soft Limit"=46, "Fault - Reverse Soft Limit"=47, "Sticky Fault - Over Temp"=48, "Sticky Fault - Under Voltage"=49, "Sticky Fault - Forward Limit"=50, "Sticky Fault - Reverse Limit"=51, "Sticky Fault - Forward Soft Limit"=52, "Sticky Fault - Reverse Soft Limit"=53, "Applied Throttle"=61, "Closed-Loop Error"=62, "Select Feedback Device"=63, "Reverse Closed-Loop Output"=64, "Mode Select"=65, "Profile Slot Select"=66, "Ramp Throttle"=67, "Reverse Feedback Sensor"=68, "Limit Switch Enabled"=69, "Limit Switch Closed - Forward"=70, "Limit Switch Closed - Reverse"=71, "Sensor Position"=73, "Sensor Velocity"=74, "Current"=75, "Brake is Enabled"=76, "Encoder Position"=77, "Encoder Velocity"=78, "Encoder Index Rise Events"=79, "Encoder A Pin State"=80, "Encoder B Pin State"=81, "Encoder Index Pin State"=82, "Analog In with Overflow"=83, "Analog In Velocity"=84, "Temperature"=85, "Battery Voltage"=86, "Reset Count"=87, "Reset Flags"=88, "Firmware Version"=89, "Settings Changed"=90] ("Parameter")
          n81 = call <vilib>:"CTRE_CANTalonSRX_RequestParameter.vi"("Parameter"=w231, "CAN Talon SRX Ref"=w228) -> ()  [unwired: 7 in, 3 out]
          n82 = call <vilib>:"CTRE_CANTalonSRX_RequestParameter.vi"("Parameter"=w230, "CAN Talon SRX Ref"=w228) -> ()  [unwired: 7 in, 3 out]
          n83 = call <vilib>:"CTRE_CANTalonSRX_RequestParameter.vi"("Parameter"=w234, "CAN Talon SRX Ref"=w228) -> ()  [unwired: 7 in, 3 out]
          n84 = call <vilib>:"CTRE_CANTalonSRX_RequestParameter.vi"("Parameter"=w232, "CAN Talon SRX Ref"=w228) -> ()  [unwired: 7 in, 3 out]
          n85 = call <vilib>:"CTRE_CANTalonSRX_RequestParameter.vi"("Parameter"=w233, "CAN Talon SRX Ref"=w228) -> ()  [unwired: 7 in, 3 out]
          n86 = call <vilib>:"CTRE_CANTalonSRX_RequestParameter.vi"("error in (no error)"=w229, "Parameter"=w236, "CAN Talon SRX Ref"=w228) -> ("error out"=w235:errorcluster, "Code"=w227:i32)  [unwired: 6 in, 1 out]
        }
      }
      n87 = Unbundle By Name(w19) -> ("CAN.Device Number"=w20:u8)
      n88 = Number To Decimal String(number=w20) -> (decimal integer string=w22:string)  [unwired: 1 in]
      n89 = Concatenate Strings("TalonSRX " ("string"), w22, " Get PID" ("string")) -> (w13:string)
      n90 = call <vilib>:"CTRE_ErrorHandle.vi"("error in"=w25, "origin"=w13, "code"=w24) -> ("error out"=w14:errorcluster)  [unwired: 8 in]
      n91 = And Array Elements(Boolean array=w26) -> (logical AND=w18:bool)
      n92 = call <vilib>:"NetComm_CAN_CloseStreamSession.vi"("error in (no error)"=w46, "Session Handle"=w47) -> ("error out"=w28:errorcluster)  [unwired: 9 in]
      n93 = Index Array(array=w32, index=0) -> (element=w42:dbl)
      n94 = Index Array(array=w32, index=1) -> (element=w33:dbl)
      n95 = Index Array(array=w32, index=2) -> (element=w34:dbl)
      n96 = Index Array(array=w32, index=3) -> (element=w35:dbl)
      n97 = Index Array(array=w32, index=4) -> (element=w36:dbl)
      n98 = Index Array(array=w32, index=5) -> (element=w31:dbl)
      n99 = Select(t=-201, s=w18, f=0 ("Code")) -> (s? t:f=w17:i32)
      n100 = call <vilib>:"CTRE_ErrorHandle.vi"("error in"=w14, "origin"=w13, "code"=w17) -> ("error out"=w12:errorcluster)  [unwired: 8 in]
      n101 = Merge Errors(w28, w12) -> (w27:errorcluster)
    }
    frame Error {
    }
  }
  "CAN Talon SRX Ref" <- w11
  "error out" <- w9
  "F" <- w3
  "I Zone" <- w4
  "Ramp Rate" <- w5
  "P" <- w6
  "I" <- w1
  "D" <- w2
